vi "Display components.vi"(0 "XY Graph":cluster{"1D":dbl[], "1D":dbl[]}[](graph), 1 "RMS error %":dbl format="%.6f", 2 "Correlation":dbl format="%.6f", 3 "RMS history":dbl[](graph), 12 "Iterations":i32, 13 "Total iterations":i32) -> ()   [LabVIEW 2010]
panel:
  out "Slide":dbl(slide) min=0.0 max=1.0 scale=0.0..1.0 scale format="%.1f"
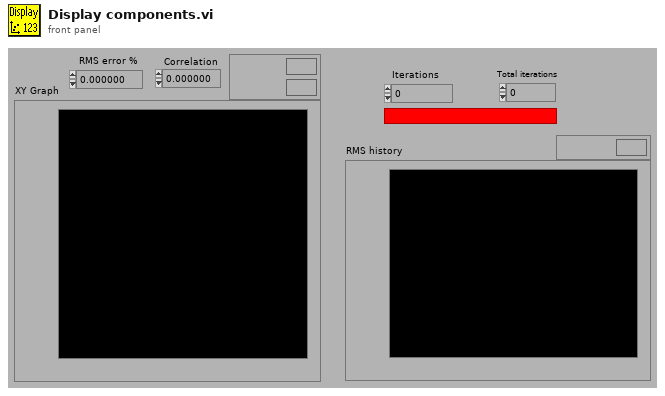
[diagram p1: front panel]
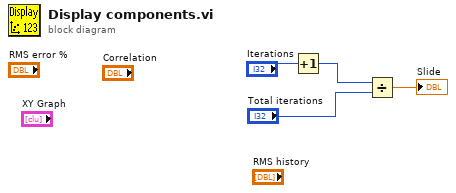
[diagram p0: block diagram]
diagram:
  n1 = Increment(x="Iterations") -> (x+1=w3:i32)
  n2 = Divide(x=w3, y="Total iterations") -> (x/y=→"Slide":dbl)
